vi "LEBITplc.IGMonitor.vi"(0 "i ref in":refnum<vi>, 1 "data":i8[](array[numeric]), 2 "i attribute in":T1, 3 "index":i32, 4 "NickNames":string, 5 "error in":errorcluster, 7 "no link":bool) -> (14 "i ref out":refnum<vi>, 15 "Data":dbl[](array[numeric]), 16 "i attribute out":T1, 17 "Indexs":i32[](array[numeric]), 19 "error out":errorcluster)   [LabVIEW 2014, in "LEBITplc.lvlib"]
uses:
  LEBITplc.lvlib
  LEBITplc.i attribute.ctl
panel:
  out "No Link":bool
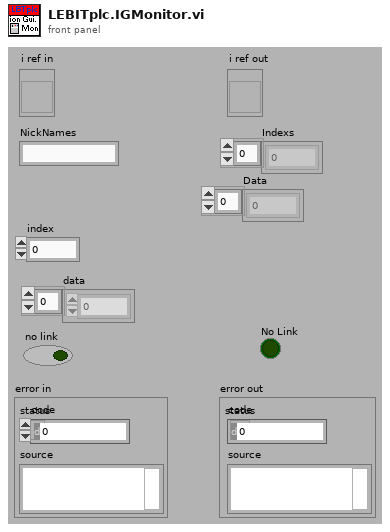
[diagram p1: front panel]
types:
  T1 = typedef "LEBITplc.lvlib/LEBITplc.i attribute.ctl" = cluster{"LLFLocation":string, "SetFileLocation":string, "nickNames":string[], "setValuePLCServiceID":i32[], "GUIServiceID":i32[], "monValuePLC":string[], "SetValueServiceID":i32[], "MonValueServiceID":i32[], "SetValue":dbl[][], "SetValueMin":dbl[], "SetValueMax":dbl[], "SetValueInfoServiceID":i32[], "GUINames":string[], "ListOfBases":string[], "Scale":dbl[], "Offset":dbl[], "setValuePLC":string[], "BaseName":string[], "ScaleServiceID":i32[], "OffsetServiceID":i32[], "AllPLCValues":string[], "CondSpecialArray":string[][], "CondSpecialIndex":i32[], "CondSpecialMonValue":dbl[], "RecentlyChanged":i32[], "SetFileLocationID":i32, "Dependent-Monitors":string[][], "LastLoadedFiles":string[], "IonGuideCalibLocation":string, "Monitor Dependent":string[], "Special":string[], "PLC?":bool[], "Start Date":string, "ListOfBasesServiceID":i32, "SETRA VISA resource":refnum<visa-resource-name>}
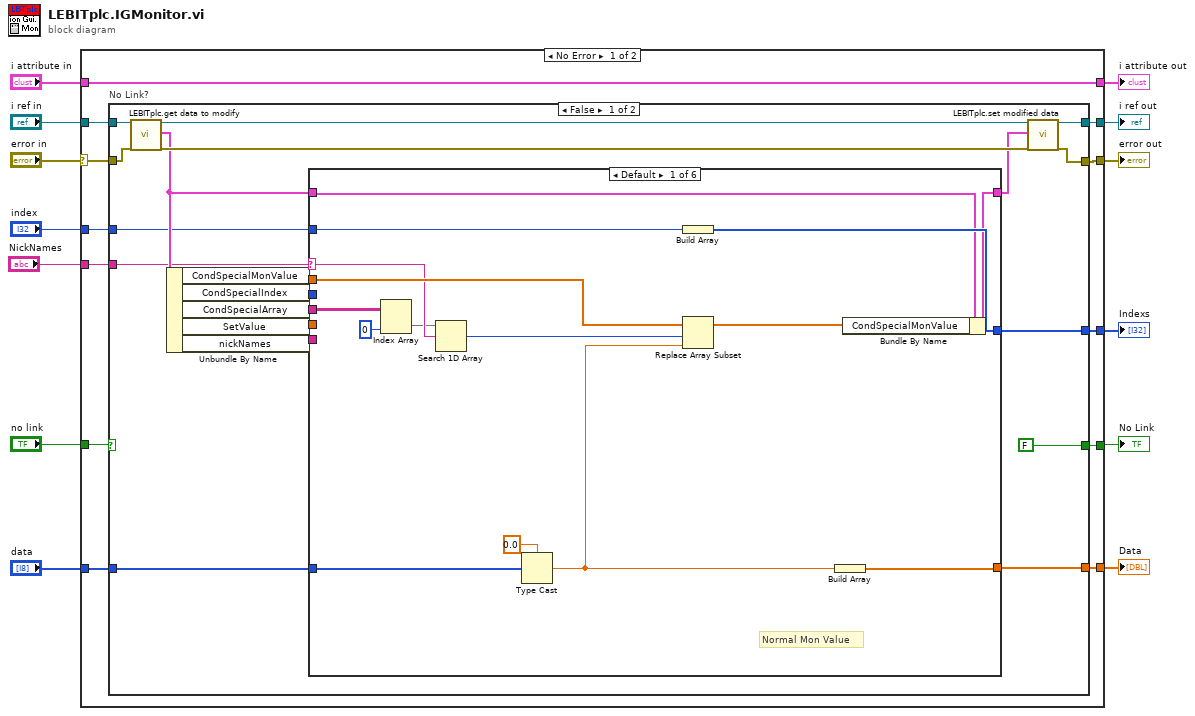
[diagram p0: block diagram]
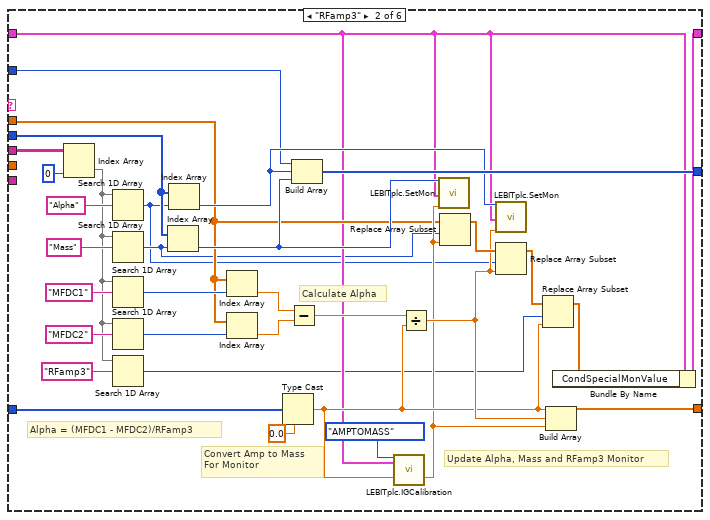
[diagram p2: hidden frame]
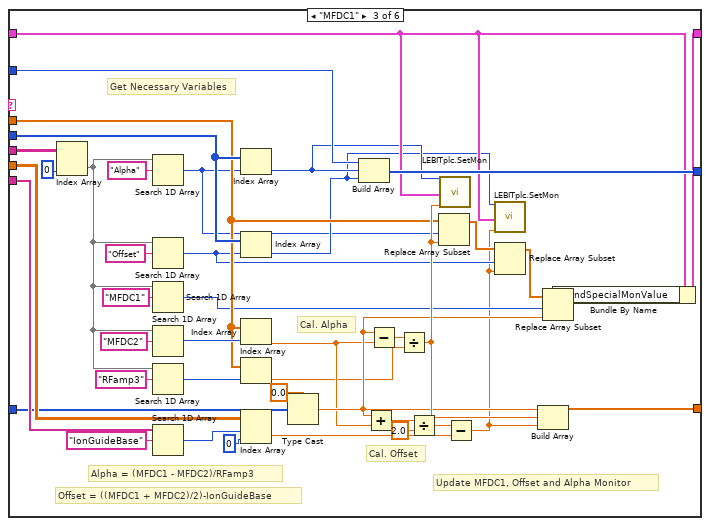
[diagram p3: hidden frame]
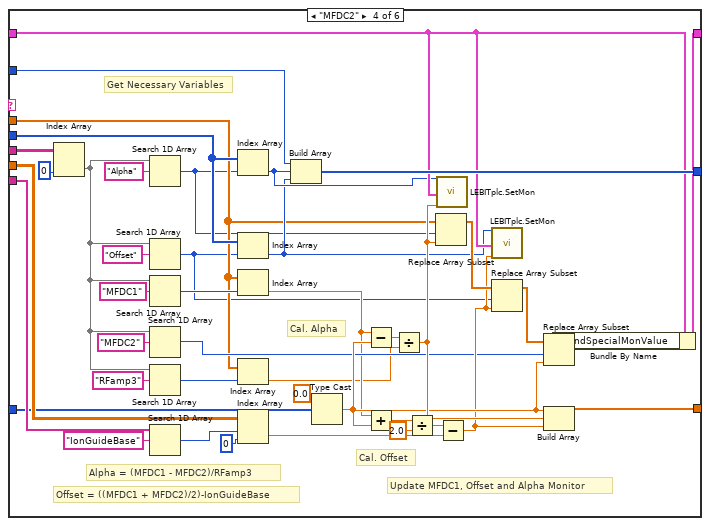
[diagram p4: hidden frame]
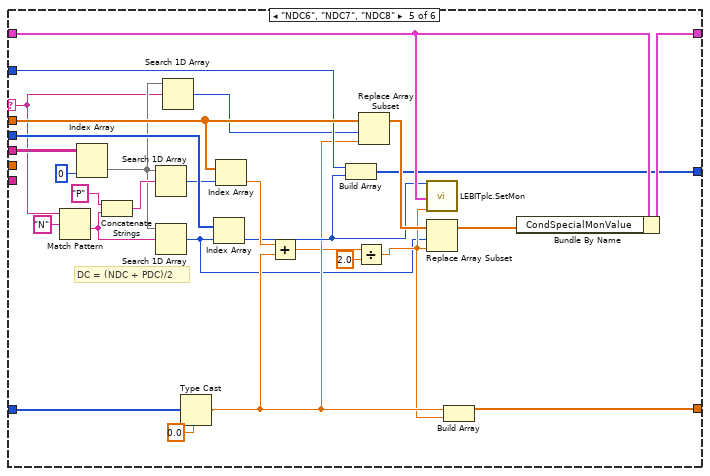
[diagram p5: hidden frame]
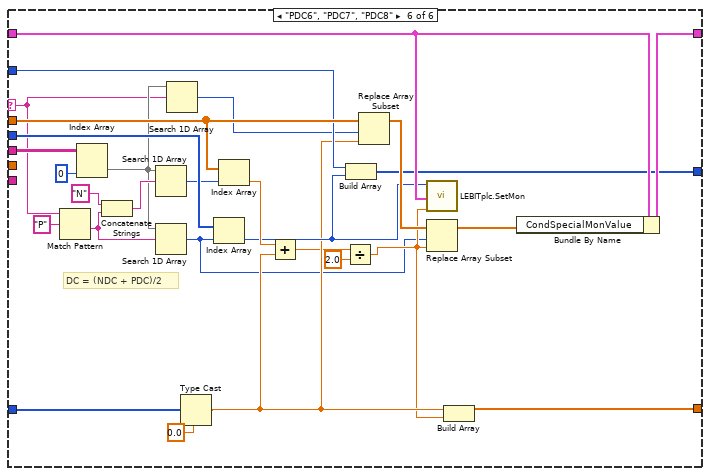
[diagram p6: hidden frame]
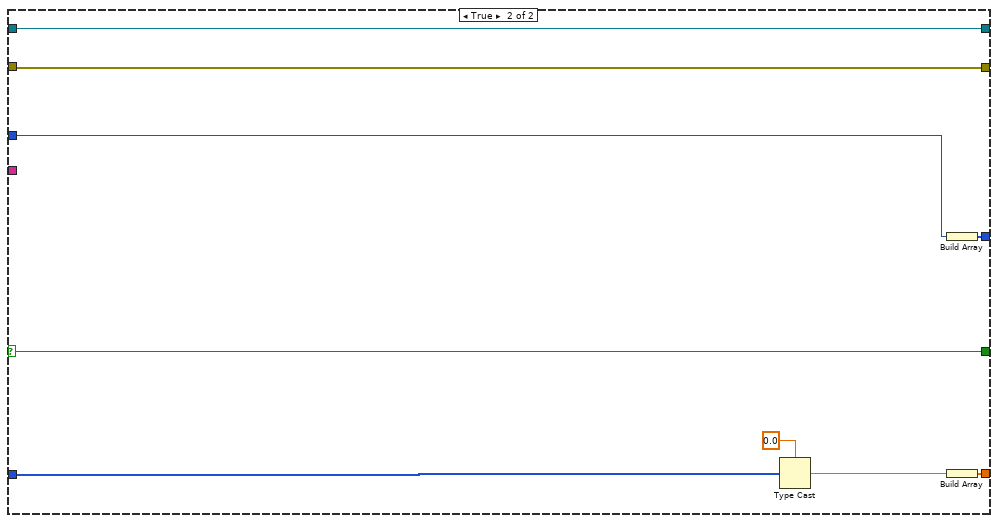
[diagram p7: hidden frame]
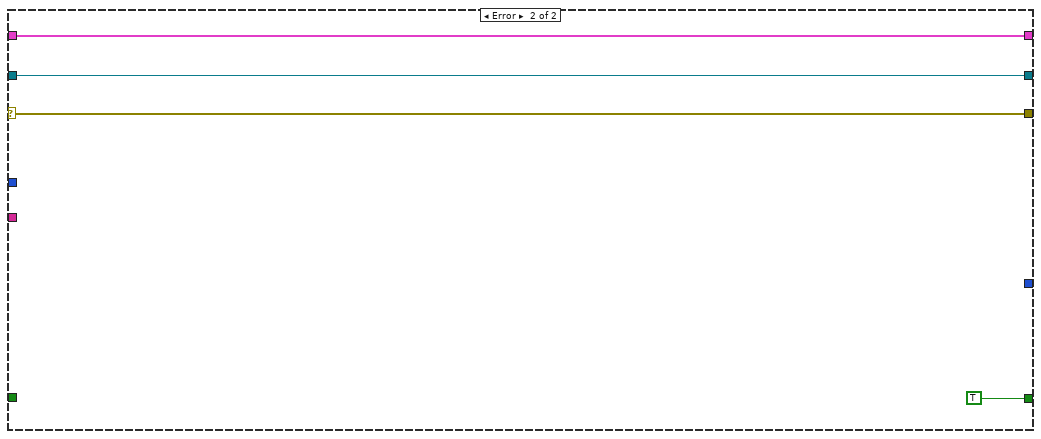
[diagram p8: hidden frame]
diagram:
  n1 = case shown="No Error" "error in" {
    selector: "error in" -> [w19 w246]
    tunnel: "NickNames" -> [w25 _]
    tunnel: [w20 w246] -> w12
    tunnel: "data" -> [w24 _]
    tunnel: "i attribute in" -> [w16 w244]
    tunnel: "i ref in" -> [w21 w245]
    tunnel: [w15 w245] -> w7
    tunnel: "index" -> [w23 _]
    tunnel: [w16 w244] -> w5
    tunnel: [w22 _] -> w4
    tunnel: "no link" -> [w18 _]
    tunnel: [w17 TRUE] -> w2
    tunnel: [w14 _] -> w1
    frame No Error {
      n2 = case "No Link?" shown="False" w18 {
        selector: w18 -> [_ w240]
        tunnel: w25 -> [w27 _]
        tunnel: w24 -> [w26 w236]
        tunnel: w23 -> [w28 w239]
        tunnel: [w44 w238] -> w22
        tunnel: w21 -> [w42 w242]
        tunnel: [w37 w242] -> w15
        tunnel: [w38 w241] -> w20
        tunnel: w19 -> [w41 w241]
        tunnel: [FALSE w240] -> w17
        tunnel: [w35 w234] -> w14
        frame False {
          n3 = call "LEBITplc.get data to modify.vi"("i ref in"=w42, "error in (no error)"=w41) -> ("i ref out"=w40:refnum<vi>, "i attribute"=w34:T1, "error out"=w39:errorcluster)  [unwired: 14 in, 1 out]
          n4 = Unbundle By Name(w34) -> ("CondSpecialMonValue"=w29:dbl[], "CondSpecialIndex"=w32:i32[], "CondSpecialArray"=w33:string[][], "SetValue"=w31:dbl[][], "nickNames"=w30:string[])
          n5 = case shown="Default" w27 {
            selector: w27 -> [w49 _ _ _ w179 w208]
            tunnel: w28 -> [w56 w63 w122 w164 w190 w218]
            tunnel: [w59 w91 w133 w175 w188 w216] -> w44
            tunnel: w34 -> [w57 w66 w123 w166 w192 w220]
            tunnel: [w58 w87 w132 w174 w191 w219] -> w36
            tunnel: [w52 w86 w128 w170 w187 w215] -> w35
            tunnel: w33 -> [w47 w80 w108 w148 w205 w233]
            tunnel: w32 -> [_ w75 w107 w149 w196 w224]
            tunnel: w31 -> [_ _ w106 w147 _ _]
            tunnel: w30 -> [_ _ w105 w146 _ _]
            tunnel: w29 -> [w50 w67 w104 w138 w195 w223]
            tunnel: w26 -> [w51 w81 w97 w145 w199 w227]
            frame Default {
              # "Normal Mon Value"
              n6 = Index Array(array=w47, index (col)=0 ("disabled index (col)")) -> (element=w46:string[])  [unwired: 1 in]
              n7 = Search 1D Array(1D array=w46, element=w49) -> (index of element=w45:i32)  [unwired: 1 in]
              n8 = Type Cast(type=0.0 ("y"), x=w51) -> (*(type *) &x=w53:dbl)
              n9 = Build Array(w56) -> (w59:i32[])
              n10 = Replace Array Subset(array=w50, new element=w53, index=w45) -> (w55:dbl[])
              n11 = Build Array(w53) -> (w52:dbl[])
              n12 = Bundle By Name(cluster=w57, "CondSpecialMonValue"=w55) -> (w58:T1)
            }
            frame "RFamp3" {
              # "Alpha = (MFDC1 - MFDC2)/RFamp3"
              # "Convert Amp to Mass \nFor Monitor"
              # "Calculate Alpha"
              # "Update Alpha, Mass and RFamp3 Monitor"
              n13 = Index Array(array=w80, index (col)=0 ("disabled index (col)")) -> (element=w61:string[])  [unwired: 1 in]
              n14 = Search 1D Array(1D array=w61, element="Alpha") -> (index of element=w64:i32)  [unwired: 1 in]
              n15 = Search 1D Array(1D array=w61, element="Mass") -> (index of element=w65:i32)  [unwired: 1 in]
              n16 = Search 1D Array(1D array=w61, element="MFDC1") -> (index of element=w73:i32)  [unwired: 1 in]
              n17 = Search 1D Array(1D array=w61, element="MFDC2") -> (index of element=w70:i32)  [unwired: 1 in]
              n18 = Search 1D Array(1D array=w61, element="RFamp3") -> (index of element=w60:i32)  [unwired: 1 in]
              n19 = Index Array(array=w75, index=w65) -> (element=w74:i32)
              n20 = Index Array(array=w75, index=w64) -> (element=w77:i32)
              n21 = Index Array(array=w67, index=w73) -> (element=w69:dbl)
              n22 = Index Array(array=w67, index=w70) -> (element=w68:dbl)
              n23 = Type Cast(type=0.0 ("y"), x=w81) -> (*(type *) &x=w84:dbl)
              n24 = Subtract(x=w69, y=w68) -> (x-y=w92:dbl)
              n25 = Build Array(w63, w77, w74) -> (w91:i32[])
              n26 = call "LEBITplc.IGCalibration.vi"("Enum"=enum16{"DelayedDC", "MASSTOAMP", "AMPTOMASS"}."AMPTOMASS", "i attribute"=w66, "AMP"=w84) -> ("MASS"=w83:dbl)  [unwired: 14 in, 2 out]
              n27 = Divide(x=w92, y=w84) -> (x/y=w85:dbl)
              n28 = call "LEBITplc.SetMon.vi"("index of element"=w74, "i attribute in"=w66, "Data"=w83) -> ()  [unwired: 17 in]
              n29 = Replace Array Subset(array=w67, new element=w83, index=w65) -> (w90:dbl[])
              n30 = call "LEBITplc.SetMon.vi"("index of element"=w77, "i attribute in"=w66, "Data"=w85) -> ()  [unwired: 17 in]
              n31 = Replace Array Subset(array=w90, new element=w85, index=w64) -> (w89:dbl[])
              n32 = Replace Array Subset(array=w89, new element=w84, index=w60) -> (w88:dbl[])
              n33 = Build Array(w84, w85, w83) -> (w86:dbl[])
              n34 = Bundle By Name(cluster=w66, "CondSpecialMonValue"=w88) -> (w87:T1)
            }
            frame "MFDC1" {
              # "Offset = ((MFDC1 + MFDC2)/2)-IonGuideBase"
              # "Alpha = (MFDC1 - MFDC2)/RFamp3"
              # "Get Necessary Variables"
              # "Cal. Offset"
              # "Cal. Alpha"
              # "Update MFDC1, Offset and Alpha Monitor"
              n35 = Index Array(array=w108, index (col)=0 ("index (row)")) -> (element=w114:string[])  [unwired: 1 in]
              n36 = Search 1D Array(1D array=w114, element="Alpha") -> (index of element=w95:i32)  [unwired: 1 in]
              n37 = Search 1D Array(1D array=w114, element="Offset") -> (index of element=w96:i32)  [unwired: 1 in]
              n38 = Search 1D Array(1D array=w114, element="MFDC1") -> (index of element=w98:i32)  [unwired: 1 in]
              n39 = Search 1D Array(1D array=w114, element="MFDC2") -> (index of element=w116:i32)  [unwired: 1 in]
              n40 = Search 1D Array(1D array=w114, element="RFamp3") -> (index of element=w117:i32)  [unwired: 1 in]
              n41 = Search 1D Array(1D array=w105, element="IonGuideBase") -> (index of element=w119:i32)  [unwired: 1 in]
              n42 = Index Array(array=w107, index=w95) -> (element=w100:i32)
              n43 = Index Array(array=w107, index=w96) -> (element=w99:i32)
              n44 = Index Array(array=w104, index=w116) -> (element=w102:dbl)
              n45 = Index Array(array=w104, index=w117) -> (element=w101:dbl)
              n46 = Index Array(array=w106, index (row)=w119, index (col)=0 ("disabled index (col)")) -> (element=w103:dbl)
              n47 = Type Cast(type=0.0 ("y"), x=w97) -> (*(type *) &x=w124:dbl)
              n48 = Build Array(w122, w100, w99) -> (w133:i32[])
              n49 = Add(x=w124, y=w102) -> (x+y=w127:dbl)
              n50 = Subtract(x=w124, y=w102) -> (x-y=w134:dbl)
              n51 = Divide(x=w134, y=w101) -> (x/y=w125:dbl)
              n52 = Divide(x=w127, y=2.0) -> (x/y=w121:dbl)
              n53 = Replace Array Subset(array=w104, new element=w125, index=w95) -> (w131:dbl[])
              n54 = call "LEBITplc.SetMon.vi"("index of element"=w100, "i attribute in"=w123, "Data"=w125) -> ()  [unwired: 17 in]
              n55 = Subtract(x=w121, y=w103) -> (x-y=w94:dbl)
              n56 = call "LEBITplc.SetMon.vi"("index of element"=w99, "i attribute in"=w123, "Data"=w94) -> ()  [unwired: 17 in]
              n57 = Replace Array Subset(array=w131, new element=w94, index=w96) -> (w130:dbl[])
              n58 = Build Array(w124, w125, w94) -> (w128:dbl[])
              n59 = Replace Array Subset(array=w130, new element=w124, index=w98) -> (w129:dbl[])
              n60 = Bundle By Name(cluster=w123, "CondSpecialMonValue"=w129) -> (w132:T1)
            }
            frame "MFDC2" {
              # "Offset = ((MFDC1 + MFDC2)/2)-IonGuideBase"
              # "Alpha = (MFDC1 - MFDC2)/RFamp3"
              # "Get Necessary Variables"
              # "Cal. Offset"
              # "Cal. Alpha"
              # "Update MFDC1, Offset and Alpha Monitor"
              n61 = Index Array(array=w148, index (col)=0 ("index (row)")) -> (element=w155:string[])  [unwired: 1 in]
              n62 = Search 1D Array(1D array=w155, element="Alpha") -> (index of element=w137:i32)  [unwired: 1 in]
              n63 = Search 1D Array(1D array=w155, element="Offset") -> (index of element=w136:i32)  [unwired: 1 in]
              n64 = Search 1D Array(1D array=w155, element="MFDC1") -> (index of element=w158:i32)  [unwired: 1 in]
              n65 = Search 1D Array(1D array=w155, element="MFDC2") -> (index of element=w143:i32)  [unwired: 1 in]
              n66 = Search 1D Array(1D array=w155, element="RFamp3") -> (index of element=w157:i32)  [unwired: 1 in]
              n67 = Search 1D Array(1D array=w146, element="IonGuideBase") -> (index of element=w160:i32)  [unwired: 1 in]
              n68 = Index Array(array=w149, index=w137) -> (element=w140:i32)
              n69 = Index Array(array=w149, index=w136) -> (element=w139:i32)
              n70 = Index Array(array=w138, index=w158) -> (element=w142:dbl)
              n71 = Index Array(array=w138, index=w157) -> (element=w141:dbl)
              n72 = Index Array(array=w147, index (row)=w160, index (col)=0 ("disabled index (col)")) -> (element=w144:dbl)
              n73 = Build Array(w164, w140, w139) -> (w175:i32[])
              n74 = Type Cast(type=0.0 ("y"), x=w145) -> (*(type *) &x=w165:dbl)
              n75 = Subtract(x=w142, y=w165) -> (x-y=w176:dbl)
              n76 = Add(x=w142, y=w165) -> (x+y=w168:dbl)
              n77 = Divide(x=w176, y=w141) -> (x/y=w167:dbl)
              n78 = Divide(x=w168, y=2.0) -> (x/y=w162:dbl)
              n79 = Replace Array Subset(array=w138, new element=w167, index=w137) -> (w173:dbl[])
              n80 = call "LEBITplc.SetMon.vi"("index of element"=w140, "i attribute in"=w166, "Data"=w167) -> ()  [unwired: 17 in]
              n81 = Subtract(x=w162, y=w144) -> (x-y=w163:dbl)
              n82 = call "LEBITplc.SetMon.vi"("index of element"=w139, "i attribute in"=w166, "Data"=w163) -> ()  [unwired: 17 in]
              n83 = Replace Array Subset(array=w173, new element=w163, index=w136) -> (w172:dbl[])
              n84 = Replace Array Subset(array=w172, new element=w165, index=w143) -> (w171:dbl[])
              n85 = Build Array(w165, w167, w163) -> (w170:dbl[])
              n86 = Bundle By Name(cluster=w166, "CondSpecialMonValue"=w171) -> (w174:T1)
            }
            frame "NDC6", "NDC7", "NDC8" {
              # "DC = (NDC + PDC)/2"
              n87 = Match Pattern(string=w179, regular expression="N") -> (after substring=w197:string)  [unwired: 1 in, 3 out]
              n88 = Index Array(array=w205, index (col)=0 ("disabled index (col)")) -> (element=w180:string[])  [unwired: 1 in]
              n89 = Concatenate Strings("P" ("string"), w197) -> (w201:string)
              n90 = Search 1D Array(1D array=w180, element=w201) -> (index of element=w181:i32)  [unwired: 1 in]
              n91 = Search 1D Array(1D array=w180, element=w197) -> (index of element=w182:i32)  [unwired: 1 in]
              n92 = Search 1D Array(1D array=w180, element=w179) -> (index of element=w178:i32)  [unwired: 1 in]
              n93 = Type Cast(type=0.0 ("y"), x=w199) -> (*(type *) &x=w186:dbl)
              n94 = Index Array(array=w196, index=w182) -> (element=w189:i32)
              n95 = Index Array(array=w195, index=w181) -> (element=w198:dbl)
              n96 = Add(x=w198, y=w186) -> (x+y=w185:dbl)
              n97 = Build Array(w190, w189) -> (w188:i32[])
              n98 = Divide(x=w185, y=2.0) -> (x/y=w184:dbl)
              n99 = Replace Array Subset(array=w195, new element=w186, index=w178) -> (w194:dbl[])
              n100 = call "LEBITplc.SetMon.vi"("index of element"=w189, "i attribute in"=w192, "Data"=w184) -> ()  [unwired: 17 in]
              n101 = Replace Array Subset(array=w194, new element=w184, index=w182) -> (w193:dbl[])
              n102 = Build Array(w186, w184) -> (w187:dbl[])
              n103 = Bundle By Name(cluster=w192, "CondSpecialMonValue"=w193) -> (w191:T1)
            }
            frame "PDC6", "PDC7", "PDC8" {
              # "DC = (NDC + PDC)/2"
              n104 = Match Pattern(string=w208, regular expression="P") -> (after substring=w225:string)  [unwired: 1 in, 3 out]
              n105 = Index Array(array=w233, index (col)=0 ("disabled index (col)")) -> (element=w209:string[])  [unwired: 1 in]
              n106 = Concatenate Strings("N" ("string"), w225) -> (w229:string)
              n107 = Search 1D Array(1D array=w209, element=w229) -> (index of element=w207:i32)  [unwired: 1 in]
              n108 = Search 1D Array(1D array=w209, element=w225) -> (index of element=w210:i32)  [unwired: 1 in]
              n109 = Search 1D Array(1D array=w209, element=w208) -> (index of element=w206:i32)  [unwired: 1 in]
              n110 = Type Cast(type=0.0 ("y"), x=w227) -> (*(type *) &x=w214:dbl)
              n111 = Index Array(array=w224, index=w210) -> (element=w217:i32)
              n112 = Index Array(array=w223, index=w207) -> (element=w226:dbl)
              n113 = Add(x=w226, y=w214) -> (x+y=w213:dbl)
              n114 = Divide(x=w213, y=2.0) -> (x/y=w212:dbl)
              n115 = Build Array(w218, w217) -> (w216:i32[])
              n116 = Replace Array Subset(array=w223, new element=w214, index=w206) -> (w222:dbl[])
              n117 = call "LEBITplc.SetMon.vi"("index of element"=w217, "i attribute in"=w220, "Data"=w212) -> ()  [unwired: 17 in]
              n118 = Replace Array Subset(array=w222, new element=w212, index=w210) -> (w221:dbl[])
              n119 = Build Array(w214, w212) -> (w215:dbl[])
              n120 = Bundle By Name(cluster=w220, "CondSpecialMonValue"=w221) -> (w219:T1)
            }
          }
          n121 = call "LEBITplc.set modified data.vi"("i ref in"=w40, "i attribute"=w36, "error in (no error)"=w39) -> ("i ref out"=w37:refnum<vi>, "error out"=w38:errorcluster)  [unwired: 15 in]
        }
        frame True {
          n122 = Type Cast(type=0.0, x=w236) -> (*(type *) &x=w237:dbl)
          n123 = Build Array(w239) -> (w238:i32[])
          n124 = Build Array(w237) -> (w234:dbl[])
        }
      }
    }
    frame Error {
    }
  }
  "error out" <- w12
  "i ref out" <- w7
  "i attribute out" <- w5
  "Indexs" <- w4
  "No Link" <- w2
  "Data" <- w1
